vi "Crop Video Size.vi"() -> ()   [LabVIEW 2017]
uses:
  WEISS-Ultrasound-Frame-Grabber/LabVIEW/Controls/Frame Grabber Data.ctl
  <vilib>/userdefined/High Color/IMAQdx.ctl
  <vilib>/vision/Image Controls.llb/IMAQ Image.ctl
  <vilib>/vision/Avi.llb/IMAQ AVI2 Refnum.ctl
  WEISS-Ultrasound-Frame-Grabber/LabVIEW/Controls/Rigid Body Info.ctl
  WEISS-Ultrasound-Frame-Grabber/LabVIEW/Controls/Position.ctl
  WEISS-Ultrasound-Frame-Grabber/LabVIEW/Controls/Orientation.ctl
  WEISS-Ultrasound-Frame-Grabber/LabVIEW/Controls/Refnums.ctl
  WEISS-Ultrasound-Frame-Grabber/LabVIEW/Controls/Recording Settings.ctl
  WEISS-Ultrasound-Frame-Grabber/LabVIEW/Controls/Operator Settings.ctl
  WEISS-Ultrasound-Frame-Grabber/LabVIEW/Controls/Operator.ctl
  WEISS-Ultrasound-Frame-Grabber/LabVIEW/Controls/Dimensions.ctl
  WEISS-Ultrasound-Frame-Grabber/LabVIEW/Controls/Room Dimensions.ctl
  <vilib>/vision/NI_Vision_Development_Module.lvlib
panel:
  in  "Codec":u16(ring)=3 items=["Cinepak Codec by Radius", "Intel IYUV codec", "Microsoft Video 1", "FF Video Codec 1 (FFV1) (NI Vision)", "Motion JPEG (NI Vision)", "Y800 Uncompressed Grey Scale (NI Vision)", "YUV 4:2:0 Planar (NI Vision)"]
  out "Saving":bool
  in  "Display?":bool
  in  "Crop":bool
  in  "Reset Crop":bool
  in  "Stop":bool
  out "Video path":path
  out "Crop ROI":i32[](array[numeric])
  in  "Frame Grabber Data":T1={"Camera Session"="", "Frame"=refnum, "AVI Refnum"=refnum, "Codecs"=[], "Frame number"=0, "Tracking File Refnum"=refnum, "Tick Count"=0, "Probe Object"=refnum, "Playback Probe Data"=[], "Rigid Body"={"Position"={"x (mm)"=0.0, "y (mm)"=0.0, "z (mm)"=0.0}, "Orientation"={"Pitch (rad)"=0.0, "Yaw (rad)"=0.0, "Roll (rad)"=0.0}, "Quaternion"={"qx"=0.0, "qy"=0.0, "qz"=0.0, "qw"=0.0}, "Tracked?"=FALSE}, "Total no frames playback"=0, "Video FPS"=0.0, "Camera connected?"=FALSE, "Scene"=refnum, "Cropped Frame"=refnum, "Tracker FPS"=0.0, "Crop ROI"=[], "Presentation Values"=[], "Elapsed time (ms)"=0, "Camera frames playback"=0, "Refnums"={"Live Refnum"=refnum, "Record Refnum"=refnum, "Recording Settings Refnum"=refnum, "Playback Refnum"=refnum, "Frame Slider Refnum"=refnum, "Pause Refnum"=refnum, "Home Refnum"=refnum, "Crop Refnum"=refnum, "Clear Crop Refnum"=refnum, "stop refnum"=refnum, "Playback Rate Refnum"=refnum, "Operator Settings Refnums"=refnum, "Presentation Refnum"=refnum, "Gestation Refnum"=refnum, "Connection Settings Refnum"=refnum}, "Dimensions"={"Probe Dimensions"={"Probe Width"=0.0, "Probe Depth"=1.0, "Probe Height"=0.0}, "Room Dimensions"={"Room Width"=0.0, "Room Depth"=0.0, "Room Height"=0.0}}}
  in  "Save":bool
  in  "Open":bool
  out "Frame":T3(plugin-control)
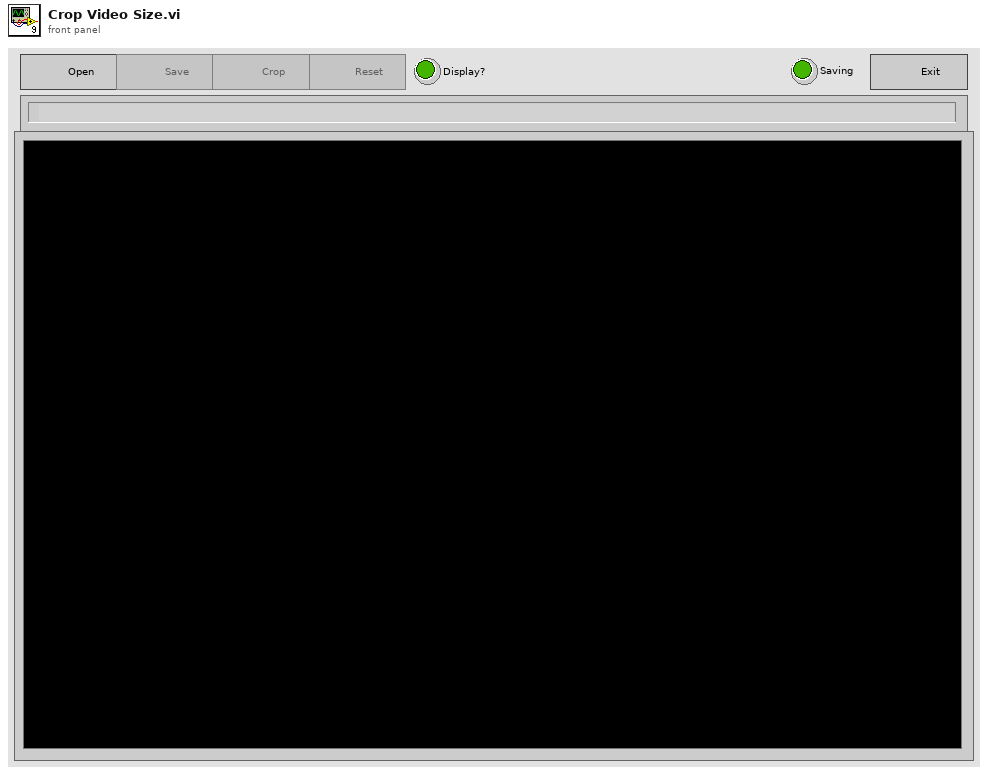
[diagram p1: front panel]
types:
  T1 = typedef "Frame Grabber Data.ctl" = cluster{"Camera Session":T2, "Frame":T3, "AVI Refnum":T4, "Codecs":string[], "Frame number":u32, "Tracking File Refnum":refnum<file>, "Tick Count":u32, "Probe Object":refnum<vi>, "Playback Probe Data":dbl[][], "Rigid Body":T5, "Total no frames playback":i32, "Video FPS":dbl, "Camera connected?":bool, "Scene":refnum<vi>, "Cropped Frame":T3, "Tracker FPS":dbl, "Crop ROI":i32[], "Presentation Values":string[], "Elapsed time (ms)":u32, "Camera frames playback":u32, "Refnums":T8, "Dimensions":T9}
  T2 = typedef "IMAQdx.ctl" = refnum<k21>
  T3 = typedef "IMAQ Image.ctl" = refnum<image>
  T4 = typedef "IMAQ AVI2 Refnum.ctl" = refnum<k20>
  T5 = typedef "Rigid Body Info.ctl" = cluster{"Position":T6, "Orientation":T7, "Quaternion":cluster{"qx":sgl, "qy":sgl, "qz":sgl, "qw":sgl}, "Tracked?":bool}
  T6 = typedef "Position.ctl" = cluster{"x (mm)":sgl, "y (mm)":sgl, "z (mm)":sgl}
  T7 = typedef "Orientation.ctl" = cluster{"Pitch (rad)":sgl, "Yaw (rad)":sgl, "Roll (rad)":sgl}
  T8 = typedef "Refnums.ctl" = cluster{"Live Refnum":refnum<vi>, "Record Refnum":refnum<vi>, "Recording Settings Refnum":refnum<vi>, "Playback Refnum":refnum<vi>, "Frame Slider Refnum":refnum<vi>, "Pause Refnum":refnum<vi>, "Home Refnum":refnum<vi>, "Crop Refnum":refnum<vi>, "Clear Crop Refnum":refnum<vi>, "stop refnum":refnum<vi>, "Playback Rate Refnum":refnum<vi>, "Operator Settings Refnums":refnum<vi>, "Presentation Refnum":refnum<vi>, "Gestation Refnum":refnum<vi>, "Connection Settings Refnum":refnum<vi>}
  T9 = typedef "Dimensions.ctl" = cluster{"Probe Dimensions":cluster{"Probe Width":sgl, "Probe Depth":sgl, "Probe Height":sgl}, "Room Dimensions":T10}
  T10 = typedef "Room Dimensions.ctl" = cluster{"Room Width":dbl, "Room Depth":dbl, "Room Height":dbl}
  T11 = enum8{"Enabled", "Disabled", "Disabled and Grayed Out"}
  T12 = typedef "Image Type" = u32
  T13 = enum16{"open", "replace", "create", "open or create", "replace or create", "replace or create with confirmation"}
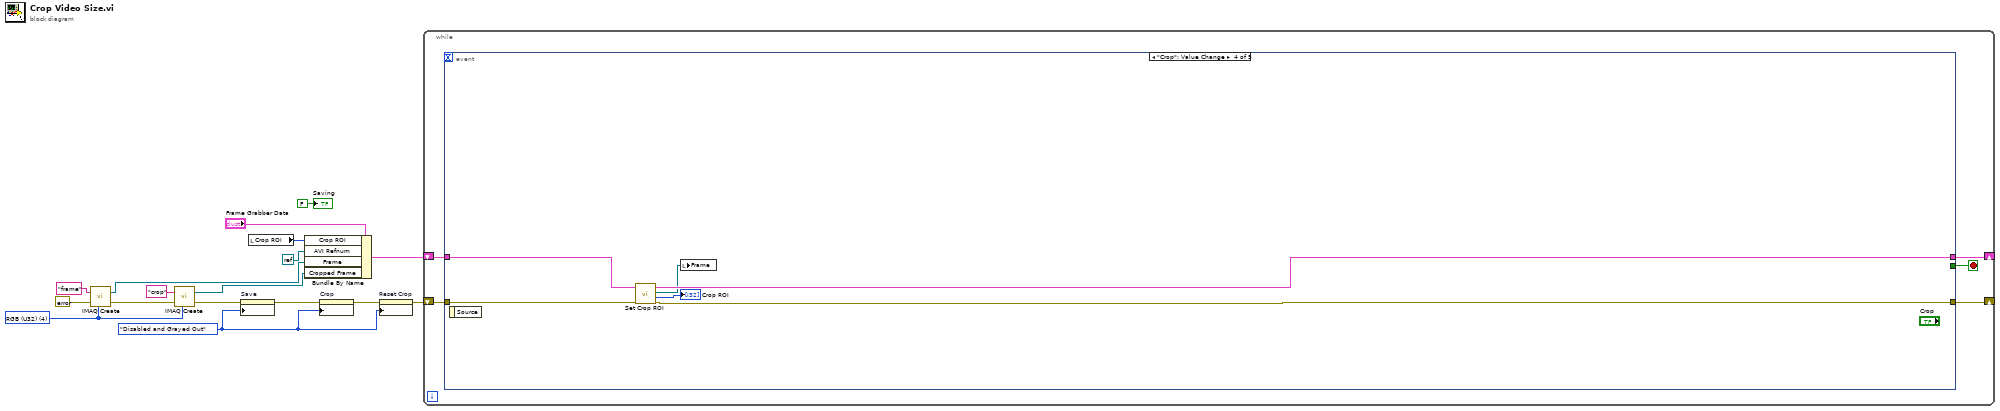
[diagram p0: block diagram]
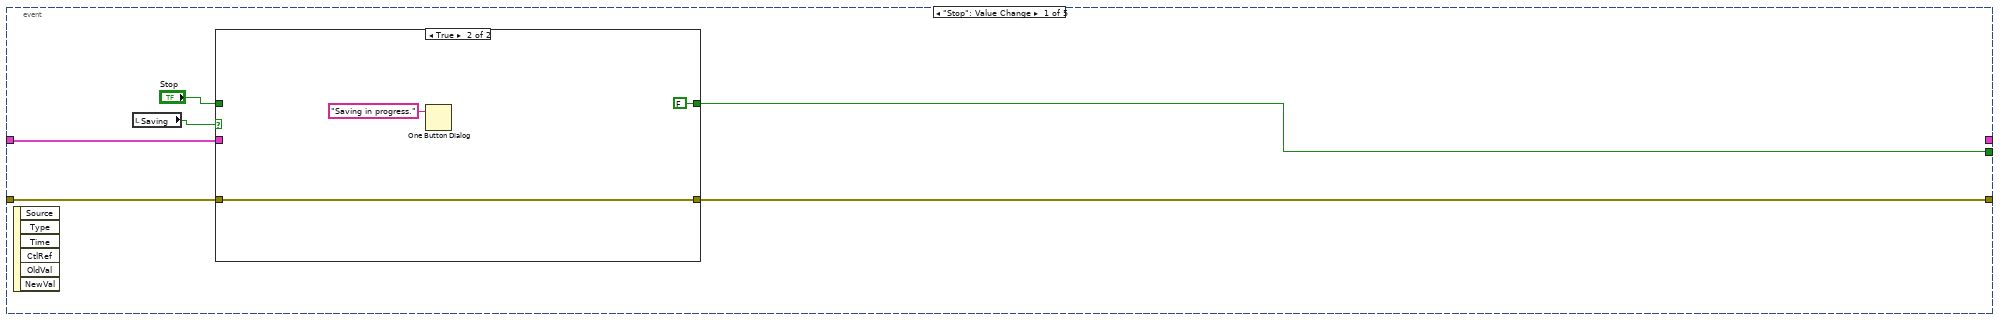
[diagram p2: hidden frame]
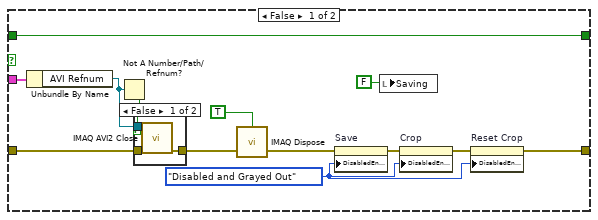
[diagram p3: hidden frame]
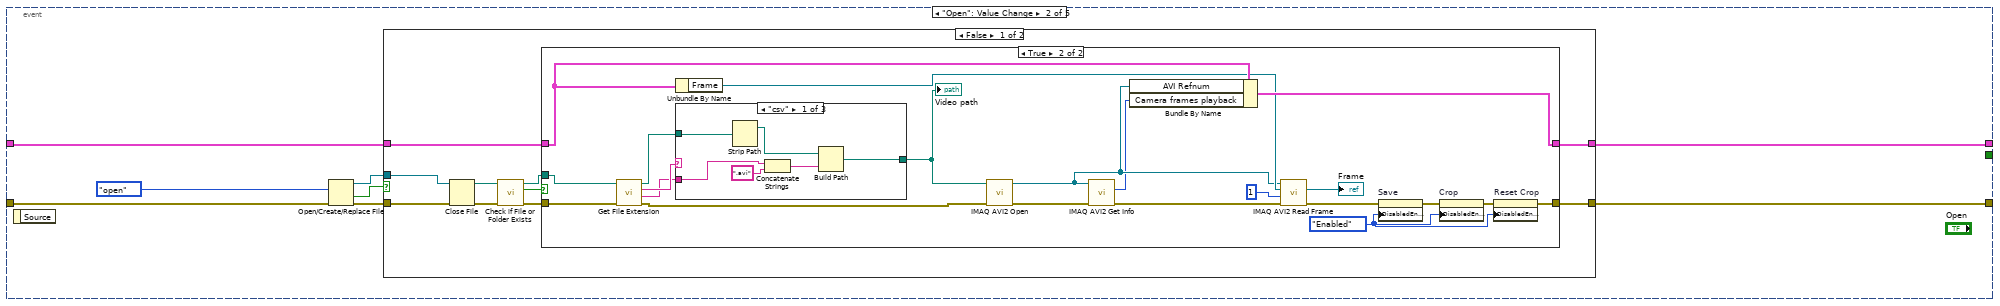
[diagram p5: hidden frame]
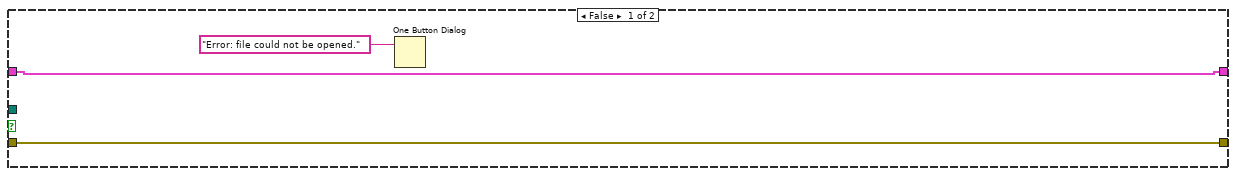
[diagram p6: hidden frame]
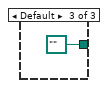
[diagram p8: hidden frame]
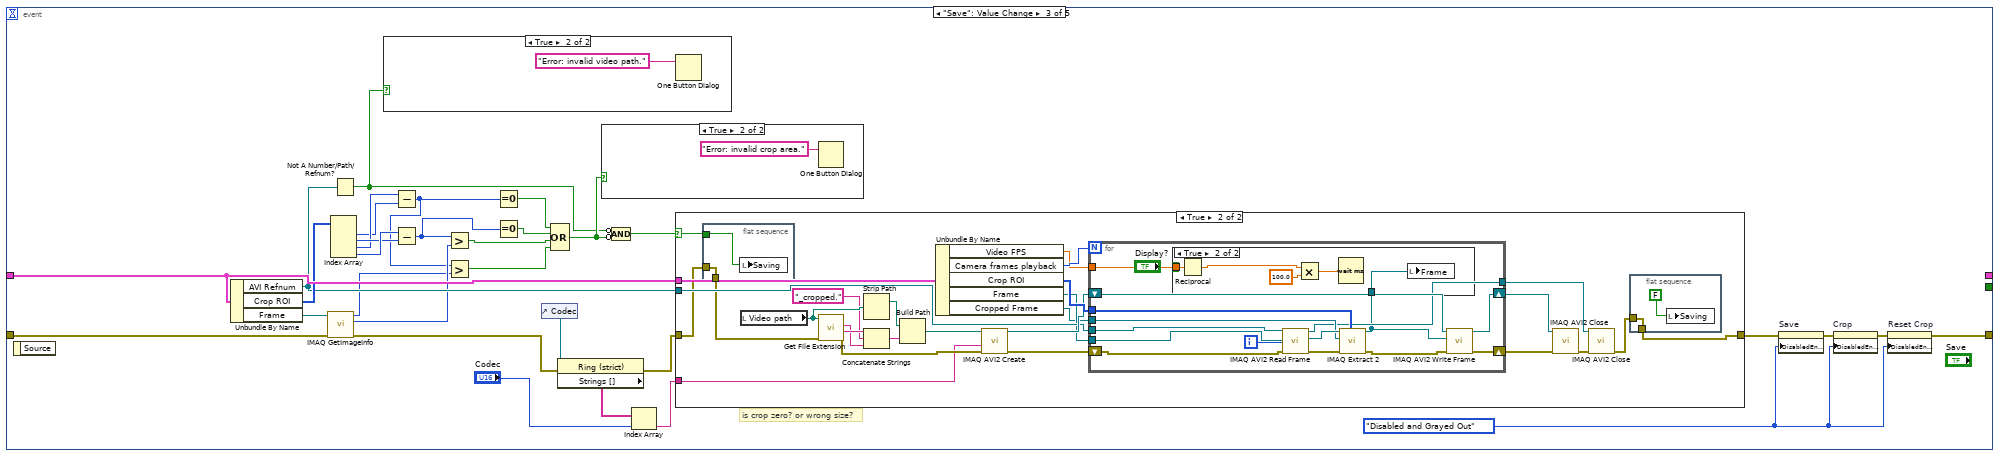
[diagram p10: hidden frame]
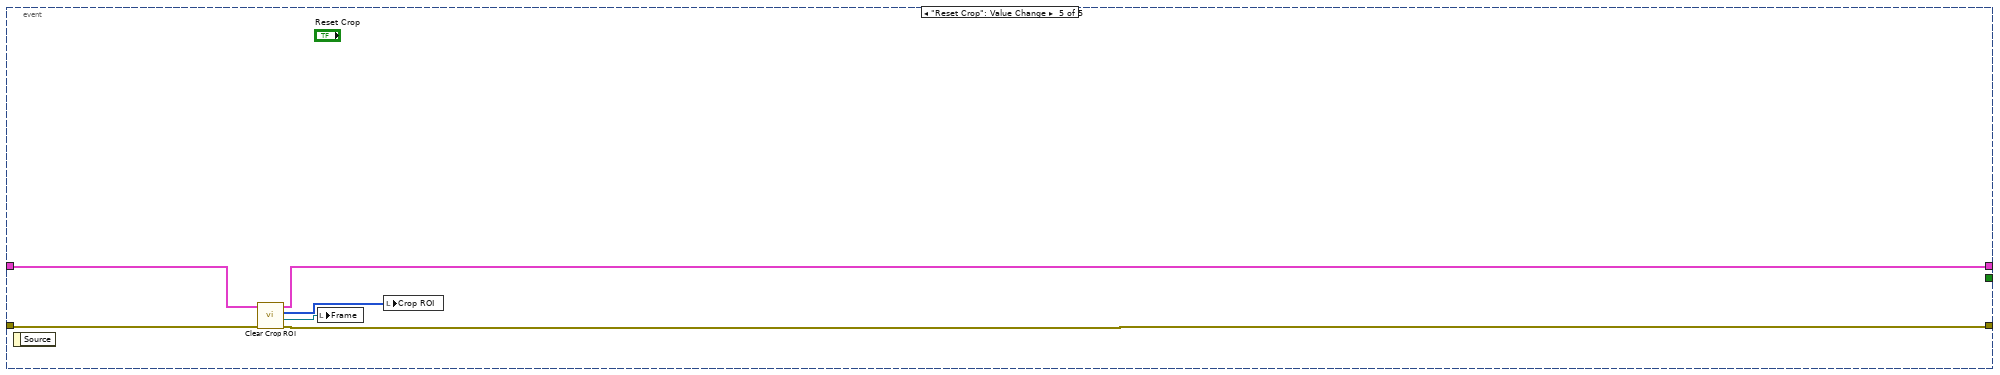
[diagram p15: hidden frame]
diagram:
  w2 = T11."Disabled and Grayed Out" ("Disabled")
  w9 = T12 4 items=["Grayscale (U8)", "Grayscale (I16)", "Grayscale (SGL)", "Complex (CSG)", "RGB (U32)", "HSL (U32)", "RGB (U64)", "Grayscale (U16)"] ("Image Type")
  n1 = call "IMAQ Create"("Image Name"="frame", "Image Type"=w9, "error in (no error)"=errorcluster {"status"=FALSE, "code"=0, "source"=""}) -> ("New Image"=w12:T3, "error out"=w10:errorcluster)  [unwired: 2 in]
  n2 = call "IMAQ Create"("Image Name"="crop", "Image Type"=w9, "error in (no error)"=w10) -> ("New Image"=w13:T3, "error out"=w6:errorcluster)  [unwired: 2 in]
  n3 = property on="Save" class="Bool"(error in=w6, "DisabledEnum"=w2) -> (error out=w5:errorcluster)  [unwired: 1 in, 1 out]
  n4 = local read "Crop ROI"() -> (w7:i32[])
  n5 = Bundle By Name(cluster="Frame Grabber Data", "Crop ROI"=w7, "AVI Refnum"=refnum<k0> refnum, "Frame"=w12, "Cropped Frame"=w13) -> (w16:T1)
  n6 = property on="Crop" class="Bool"(error in=w5, "DisabledEnum"=w2) -> (error out=w3:errorcluster)  [unwired: 1 in, 1 out]
  n7 = property on="Reset Crop" class="Bool"(error in=w3, "DisabledEnum"=w2) -> (error out=w4:errorcluster)  [unwired: 1 in, 1 out]
  n8 = while {
    shift-right: [w19] -> _
    shift-left: w16 -> [w20]
    shift-right: [w18] -> _
    shift-left: w4 -> [w21]
    stop <- w22 stop-if-true
    n9 = event shown="[3] \"Crop\": Value Change" {
      selector: _ -> [_ _ _ _ _]
      dyn-events: _ -> [_ _ _ _ _]
      timeout: _ -> [_ _ _ _ _]
      tunnel: [w23 _ _ _ _] -> w22
      tunnel: w21 -> [w28 w56 w118 w191 w195]
      tunnel: w20 -> [w27 w51 w131 w192 w198]
      tunnel: [_ w50 _ w190 w193] -> w19
      tunnel: [w26 w49 w109 w187 w194] -> w18
      event "Stop": Value Change {
        n10 = event-data() -> ()  [unwired: 1 in, 6 out]
        n11 = local read "Saving"() -> (w24:bool)
        n12 = case shown="True" w24 {
          tunnel: w28 -> [w41 w47]
          tunnel: w27 -> [w40 _]
          tunnel: [w36 w47] -> w26
          tunnel: "Stop" -> [w29 _]
          tunnel: [w29 FALSE ("Stop")] -> w23
          frame False {
            w33 = T11."Disabled and Grayed Out" ("Disabled")
            n13 = Unbundle By Name(w40) -> ("AVI Refnum"=w31:T4)
            n14 = Not A Number/Path/Refnum?(number/path/refnum=w31) -> (NaN/Path/Refnum?=w30:bool)
            n15 = case shown="False" w30 {
              tunnel: w41 -> [w44 w45]
              tunnel: [w43 w45] -> w38
              tunnel: w31 -> [w42 _]
              frame False {
                n16 = call "IMAQ AVI2 Close"("error in (no error)"=w44, "AVI Refnum"=w42) -> ("error out"=w43:errorcluster)  [unwired: 9 in]
              }
              frame True {
              }
            }
            n17 = call "IMAQ Dispose"("All Images? (No)"=TRUE, "error in (no error)"=w38) -> ("error out"=w37:errorcluster)  [unwired: 4 in]
            n18 = property on="Save" class="Bool"(error in=w37, "DisabledEnum"=w33) -> (error out=w34:errorcluster)  [unwired: 1 in, 1 out]
            n19 = local write "Saving"(FALSE) -> ()
            n20 = property on="Crop" class="Bool"(error in=w34, "DisabledEnum"=w33) -> (error out=w35:errorcluster)  [unwired: 1 in, 1 out]
            n21 = property on="Reset Crop" class="Bool"(error in=w35, "DisabledEnum"=w33) -> (error out=w36:errorcluster)  [unwired: 1 in, 1 out]
          }
          frame True {
            n22 = One Button Dialog(message="Saving in progress.") -> ()  [unwired: 1 in, 1 out]
          }
        }
      }
      event "Open": Value Change {
        n23 = event-data() -> ()  [unwired: 1 in, 1 out]
        n24 = Open/Create/Replace File(error in=w56, operation (0:open)=T13."open") -> (refnum out=w52:refnum<file>, cancelled=w55:bool, error out=w53:errorcluster)  [unwired: 4 in]
        n25 = case shown="False" w55 {
          tunnel: w53 -> [w63 w99]
          tunnel: w52 -> [w64 _]
          tunnel: w51 -> [w60 w100]
          tunnel: [w59 w100] -> w50
          tunnel: [w57 w99] -> w49
          frame False {
            n26 = Close File(refnum=w64, error in=w63) -> (path=w61:path, error out=w62:errorcluster)
            n27 = call <vilib>:"Check if File or Folder Exists.vi"("error in (no error)"=w62, "path"=w61) -> ("error out"=w66:errorcluster, "file or folder exists?"=w58:bool, "dup path"=w65:path)  [unwired: 7 in]
            n28 = case shown="True" w58 {
              tunnel: w66 -> [w68 w76]
              tunnel: w65 -> [_ w72]
              tunnel: w60 -> [w69 w89]
              tunnel: [w69 w90] -> w59
              tunnel: [w68 w78] -> w57
              frame False {
                n29 = One Button Dialog(message="Error: file could not be opened.") -> ()  [unwired: 1 in, 1 out]
              }
              frame True {
                w77 = T11."Enabled" ("Disabled")
                n30 = call <vilib>:"Get File Extension.vi"("error in (no error)"=w76, "file"=w72) -> ("error out"=w75:errorcluster, "filename without extension"=w73:string, "lowercase file extension"=w74:string, "dup file"=w71:path)  [unwired: 5 in, 1 out]
                n31 = Unbundle By Name(w89) -> ("Frame"=w88:T3)
                n32 = case shown="\"csv\"" w74 {
                  tunnel: w73 -> [w96 _ _]
                  tunnel: [w91 w97 path "" ("dup file")] -> w70
                  tunnel: w71 -> [w92 w97 _]
                  frame "csv" {
                    n33 = Strip Path(path=w92) -> (stripped path=w94:path)  [unwired: 1 out]
                    n34 = Concatenate Strings(w96, ".avi" ("string")) -> (w93:string)
                    n35 = Build Path(base path=w94, name or relative path=w93) -> (appended path=w91:path)
                  }
                  frame "avi" {
                  }
                  frame Default {
                  }
                }
                "Video path" <- w70
                n36 = call "IMAQ AVI2 Open"("error in (no error)"=w75, "AVI File Path"=w70) -> ("error out"=w84:errorcluster, "AVI Refnum"=w85:T4)  [unwired: 8 in]
                n37 = call "IMAQ AVI2 Get Info"("error in (no error)"=w84, "AVI Refnum"=w85) -> ("error out"=w83:errorcluster, "Number of Frames"=w82:u32)  [unwired: 5 in, 3 out]
                n38 = Bundle By Name(cluster=w89, "AVI Refnum"=w85, "Camera frames playback"=w82) -> (w90:T1)
                n39 = call "IMAQ AVI2 Read Frame"("error in (no error)"=w83, "Frame Number"=u32 1, "Image"=w88, "AVI Refnum"=w85) -> ("error out"=w81:errorcluster, "Image Out"=→"Frame":T3)  [unwired: 5 in, 1 out]
                n40 = property on="Save" class="Bool"(error in=w81, "DisabledEnum"=w77) -> (error out=w80:errorcluster)  [unwired: 1 in, 1 out]
                n41 = property on="Crop" class="Bool"(error in=w80, "DisabledEnum"=w77) -> (error out=w79:errorcluster)  [unwired: 1 in, 1 out]
                n42 = property on="Reset Crop" class="Bool"(error in=w79, "DisabledEnum"=w77) -> (error out=w78:errorcluster)  [unwired: 1 in, 1 out]
              }
            }
          }
          frame True {
          }
        }
      }
      event "Save": Value Change {
        w107 = T11."Disabled and Grayed Out" ("Disabled")
        # "is crop zero? or wrong size?"
        n43 = event-data() -> ()  [unwired: 1 in, 1 out]
        n44 = Unbundle By Name(w131) -> ("AVI Refnum"=w119:T4, "Crop ROI"=w124:i32[], "Frame"=w117:T3)
        n45 = call "IMAQ GetImageInfo"("error in (no error)"=w118, "Image"=w117) -> ("error out"=w106:errorcluster, "Y Resolution"=w116:i32, "X Resolution"=w114:i32)  [unwired: 2 in, 5 out]
        n46 = Index Array(array=w124) -> (element #1=w125:i32, element #2=w127:i32, element #3=w126:i32, element #4=w128:i32)  [unwired: 4 in]
        n47 = Not A Number/Path/Refnum?(number/path/refnum=w119) -> (NaN/Path/Refnum?=w120:bool)
        n48 = case shown="True" w120 {
          frame False {
          }
          frame True {
            n49 = One Button Dialog(message="Error: invalid video path.") -> ()  [unwired: 1 in, 1 out]
          }
        }
        n50 = Subtract(x=w126, y=w125) -> (x-y=w113:i32)
        n51 = Subtract(x=w128, y=w127) -> (x-y=w111:i32)
        n52 = Greater?(x=w111, y=w116) -> (0:w115:bool)
        n53 = Greater?(x=w113, y=w114) -> (0:w112:bool)
        n54 = Equal To 0?(x=w113) -> (x = 0?=w129:bool)
        n55 = Equal To 0?(x=w111) -> (x = 0?=w130:bool)
        n56 = control-ref of="Codec"() -> (w104:refnum<vi>)
        n57 = Compound Arithmetic op=OR(w129, w130, w115, w112) -> (w121:bool)
        n58 = property class="Ring (strict)"(reference=w104, error in=w106) -> (error out=w105:errorcluster, "Strings []"=w102:string[])  [unwired: 1 out]
        n59 = case shown="True" w121 {
          frame False {
          }
          frame True {
            n60 = One Button Dialog(message="Error: invalid crop area.") -> ()  [unwired: 1 in, 1 out]
          }
        }
        n61 = Compound Arithmetic op=AND(invert w120, invert w121) -> (w122:bool)
        n62 = Index Array(array=w102, index="Codec") -> (element=w101:string)
        n63 = case shown="True" w122 {
          selector: w122 -> [_ w140]
          tunnel: w131 -> [_ w161]
          tunnel: w119 -> [_ w148]
          tunnel: [w134 w136] -> w123
          tunnel: w105 -> [w134 w139]
          tunnel: w101 -> [_ w135]
          frame False {
          }
          frame True {
            n64 = flat-sequence {
              tunnel: w140 -> [w165]
              tunnel: w139 -> [w164]
              tunnel: [w164] -> w138
              frame #0 {
                n65 = local write "Saving"(w165) -> ()
              }
            }
            n66 = local read "Video path"() -> (w156:path)
            n67 = call <vilib>:"Get File Extension.vi"("error in (no error)"=w138, "file"=w156) -> ("error out"=w157:errorcluster, "filename without extension"=w154:string, "lowercase file extension"=w152:string)  [unwired: 5 in, 2 out]
            n68 = Strip Path(path=w156) -> (stripped path=w155:path)  [unwired: 1 out]
            n69 = Concatenate Strings(w154, "_cropped." ("string"), w152) -> (w151:string)
            n70 = Build Path(base path=w155, name or relative path=w151) -> (appended path=w150:path)
            n71 = Unbundle By Name(w161) -> ("Video FPS"=w141:dbl, "Camera frames playback"=w160:u32, "Crop ROI"=w159:i32[], "Frame"=w147:T3, "Cropped Frame"=w146:T3)
            n72 = call "IMAQ AVI2 Create"("error in (no error)"=w157, "Codec"=w135, "AVI Path"=w150) -> ("error out"=w149:errorcluster, "AVI Refnum"=w158:T4)  [unwired: 7 in]
            n73 = for {
              N: w160 -> [_]
              shift-right: [w176] -> w145
              shift-left: w149 -> [w180]
              tunnel: w159 -> [w179]
              tunnel: w148 -> [w175]
              tunnel: w147 -> [w174]
              tunnel: w146 -> [w172]
              shift-right: [w171] -> w144
              shift-left: w158 -> [w178]
              tunnel: [w170] -> w142
              tunnel: w141 -> [w167]
              i -> [w181]
              n74 = call "IMAQ AVI2 Read Frame"("error in (no error)"=w180, "Frame Number"=w181, "Image"=w174, "AVI Refnum"=w175) -> ("error out"=w168:errorcluster, "Image Out"=w173:T3, "AVI Refnum (duplicate)"=w170:T4)  [unwired: 5 in]
              n75 = call "IMAQ Extract 2"("Optional Rectangle"=w179, "error in (no error)"=w168, "Image Dst"=w172, "Image Src"=w173) -> ("error out"=w177:errorcluster, "Image Dst Out"=w169:T3)  [unwired: 6 in]
              n76 = case shown="True" "Display?" {
                tunnel: w169 -> [_ w186]
                tunnel: w167 -> [_ w185]
                frame False {
                }
                frame True {
                  n77 = Reciprocal(x=w185) -> (1/x=w184:dbl)
                  n78 = Multiply(x=w184, y=100.0) -> (x*y=w182:dbl)
                  n79 = Wait (ms)(milliseconds to wait=w182) -> ()  [unwired: 1 out]
                  n80 = local write "Frame"(w186) -> ()
                }
              }
              n81 = call "IMAQ AVI2 Write Frame"("error in (no error)"=w177, "Image"=w169, "AVI Refnum"=w178) -> ("error out"=w176:errorcluster, "AVI Refnum (duplicate)"=w171:T4)  [unwired: 6 in, 1 out]
            }
            n82 = call "IMAQ AVI2 Close"("error in (no error)"=w145, "AVI Refnum"=w144) -> ("error out"=w143:errorcluster)  [unwired: 9 in]
            n83 = call "IMAQ AVI2 Close"("error in (no error)"=w143, "AVI Refnum"=w142) -> ("error out"=w137:errorcluster)  [unwired: 9 in]
            n84 = flat-sequence {
              tunnel: w137 -> [w163]
              tunnel: [w163] -> w136
              frame #0 {
                n85 = local write "Saving"(FALSE) -> ()
              }
            }
          }
        }
        n86 = property on="Save" class="Bool"(error in=w123, "DisabledEnum"=w107) -> (error out=w108:errorcluster)  [unwired: 1 in, 1 out]
        n87 = property on="Crop" class="Bool"(error in=w108, "DisabledEnum"=w107) -> (error out=w110:errorcluster)  [unwired: 1 in, 1 out]
        n88 = property on="Reset Crop" class="Bool"(error in=w110, "DisabledEnum"=w107) -> (error out=w109:errorcluster)  [unwired: 1 in, 1 out]
      }
      event "Crop": Value Change {
        n89 = event-data() -> ()  [unwired: 1 in, 1 out]
        n90 = call "Set Crop ROI.vi"("error in (no error)"=w191, "Frame Grabber Data in"=w192) -> ("error out"=w187:errorcluster, "Crop ROI"=→"Crop ROI":i32[], "Image Out"=w189:T3, "Frame Grabber Data out"=w190:T1)  [unwired: 6 in]
        n91 = local write "Frame"(w189) -> ()
      }
      event "Reset Crop": Value Change {
        n92 = event-data() -> ()  [unwired: 1 in, 1 out]
        n93 = call "Clear Crop ROI.vi"("error in (no error)"=w195, "Frame Grabber Data in"=w198) -> ("error out"=w194:errorcluster, "Image Out"=w197:T3, "Crop ROI"=w196:i32[], "Frame Grabber Data out"=w193:T1)  [unwired: 6 in]
        n94 = local write "Frame"(w197) -> ()
        n95 = local write "Crop ROI"(w196) -> ()
      }
    }
  }
  "Saving" <- FALSE ("Saving")
